vi "Read (Single Point).vi"(8 "error in (no error)":errorcluster, 10 "timeout [ms]":i32=10000, 11 "VISA resource name":refnum<visa-resource-name>) -> (0 "error out":errorcluster, 2 "Measurement":dbl, 3 "VISA resource name out":refnum<visa-resource-name>)   [LabVIEW 2011, in "Agilent 34401.lvlib"]
doc: "Reads and returns a single measurement from the instrument."
uses:
  Agilent 34401.lvlib
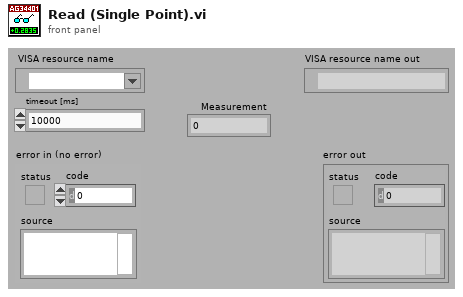
[diagram p1: front panel]
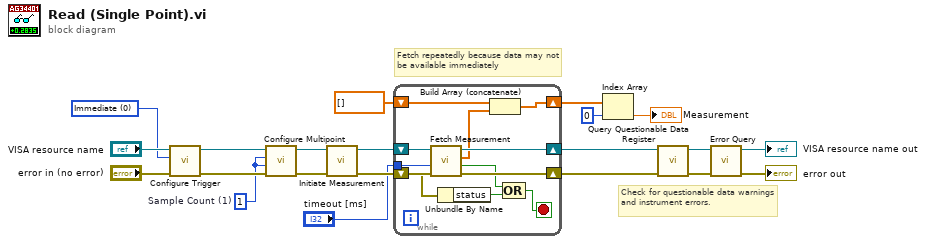
[diagram p0: block diagram]
diagram:
  w8 = u16 0 items=["Immediate", "Software (Bus)", "External", "Internal"] ("Trigger Source (0: Immediate)")
  w7 = 1  # Sample Count (1)
  # "Check for questionable data warnings and instrument errors."
  # "Fetch repeatedly because data may not be available immediately"
  n1 = call "Configure Trigger.vi"("error in (no error)"="error in (no error)", "Trigger Source (0: Immediate)"=w8, "VISA resource name"="VISA resource name") -> ("error out"=w11:errorcluster, "VISA resource name out"=w12:refnum<visa-resource-name>)  [unwired: 7 in]
  n2 = call "Configure Multipoint.vi"("error in (no error)"=w11, "Sample Count (1)"=w7, "Trigger Count (1)"=w7, "VISA resource name"=w12) -> ("error out"=w9:errorcluster, "VISA resource name out"=w10:refnum<visa-resource-name>)  [unwired: 6 in]
  n3 = call "Initiate Measurement.vi"("error in (no error)"=w9, "VISA resource name"=w10) -> ("error out"=w14:errorcluster, "VISA resource name out"=w13:refnum<visa-resource-name>)  [unwired: 8 in]
  n4 = while {
    shift-right: [w32] -> w18
    shift-left: w13 -> [w30]
    shift-right: [w29] -> w17
    shift-left: w14 -> [w31]
    shift-right: [w24] -> w15
    shift-left: dbl[] [] -> [w23]
    tunnel: "timeout [ms]" -> [w22]
    stop <- w26 stop-if-true
    n5 = call "Fetch Measurement.vi"("error in (no error)"=w31, "Timeout (10000 ms)"=w22, "VISA resource name"=w30) -> ("error out"=w29:errorcluster, "End of Data?"=w28:bool, "Measurements"=w25:dbl[], "VISA resource name out"=w32:refnum<visa-resource-name>)  [unwired: 5 in]
    n6 = Unbundle By Name(w29) -> ("status"=w27:bool)
    n7 = Build Array (concatenate)(w23, w25) -> (w24:dbl[])
    n8 = Compound Arithmetic op=OR(w28, w27) -> (w26:bool)
  }
  n9 = Index Array(array=w15, index=0) -> (element=→"Measurement":dbl)
  n10 = call "Query Questionable Data Register.vi"("error in (no error)"=w17, "VISA resource name"=w18) -> ("error out"=w5:errorcluster, "VISA resource name out"=w4:refnum<visa-resource-name>)  [unwired: 7 in, 1 out]
  n11 = call "Error Query.vi"("error in (no error)"=w5, "VISA resource name"=w4) -> ("error out"=→"error out":errorcluster, "VISA resource name out"=→"VISA resource name out":refnum<visa-resource-name>)  [unwired: 6 in, 2 out]
